vi "GenKeyBoardBlankImage.vi"(6 "KeyNumber":i32=10, 7 "WhiteKeySize":cluster{"Width":i32, "Hieght":i32}={"Width"=21, "Hieght"=147}, 8 "error in (no error)":errorcluster) -> (0 "error out":errorcluster, 3 "Image Out":T1)   [LabVIEW 2015]
uses:
  <vilib>/vision/Image Controls.llb/IMAQ Image.ctl
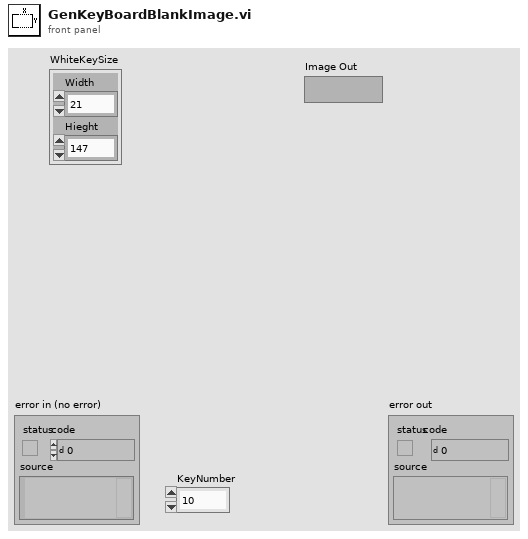
[diagram p1: front panel]
types:
  T1 = typedef "IMAQ Image.ctl" = refnum<image>
  T2 = typedef "Image Type" = u32
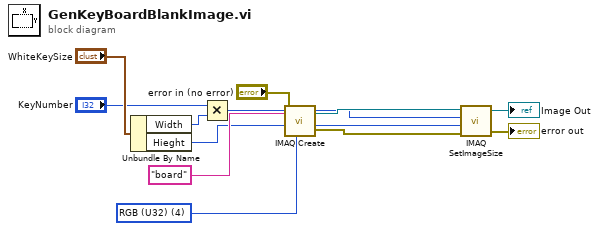
[diagram p0: block diagram]
diagram:
  w11 = T2 4 items=["Grayscale (U8)", "Grayscale (I16)", "Grayscale (SGL)", "Complex (CSG)", "RGB (U32)", "HSL (U32)", "RGB (U64)", "Grayscale (U16)"] ("Image Type")
  n1 = Unbundle By Name("WhiteKeySize") -> ("Width"=w6:i32, "Hieght"=w8:i32)
  n2 = Multiply(x="KeyNumber", y=w6) -> (x*y=w9:i32)
  n3 = call "IMAQ Create"("Image Name"="board", "Image Type"=w11, "error in (no error)"="error in (no error)") -> ("New Image"=w10:T1, "error out"=w7:errorcluster)  [unwired: 2 in]
  n4 = call "IMAQ SetImageSize"("error in (no error)"=w7, "Y Resolution"=w8, "X Resolution"=w9, "Image"=w10) -> ("error out"=→"error out":errorcluster, "Image Out"=→"Image Out":T1)  [unwired: 1 in]
